vi "小波阈值降噪—优化.vi"(5 "Tab Control":enum32{"None", "Threshold", "Levels"}(tab)=enum."Threshold", 8 "signal out":waveform(dbl)) -> (0 "Denoised Signal":waveform(dbl)(graph)={"t0"=timestamp(0 s since 1904-01-01), "dt"=0.001, "Y"=[]}, 2 "Mean Squared Error":dbl=0.019874592460755663 format="%.2f", 3 "Thresholded Wavelet \nTransform":waveform(dbl)(graph)={"t0"=timestamp(0 s since 1904-01-01), "dt"=0.001, "Y"=[]})   [LabVIEW 2015]
doc: "This LabVIEW VI demonstrates several methods of wavelet-based noise reduction using the Daubechies 4 wavelet. Although it does not require the Signal Processing Toolset, that toolset could be used to extend this demo with other types of wavelets."
uses:
  <vilib>/gmath/NI_Gmath.lvlib
  <vilib>/measure/NI_MABase.lvlib
  <vilib>/Analysis/NI_AALPro.lvlib
panel:
  in  "signal out":waveform(dbl)={"t0"=timestamp(0 s since 1904-01-01), "dt"=0.0, "Y"=[]}
  in  "Threshold":dbl=0.3400000000000002 step=0.01 format="%.2f"
  in  "Keep N Smoothest":i16=10 max=10
  in  "Continuously\nUpdate Signal?":bool
  in  "standard deviation":dbl=0.2 format="%.2f"
  in  "amplitude":dbl=1.0 format="%.2p"
  in  "frequency":dbl=10.0 format="%.2p"
  out "Original (Noise free) signal":waveform(dbl)(graph)={"t0"=timestamp(0 s since 1904-01-01), "dt"=0.001, "Y"=[]}
  out "Signal + Noise":waveform(dbl)(graph)={"t0"=timestamp(0 s since 1904-01-01), "dt"=0.001, "Y"=[]}
  out "Added Noise":waveform(dbl)(graph)={"t0"=timestamp(0 s since 1904-01-01), "dt"=0.001, "Y"=[]}
  in  "sampling info":cluster{"Fs":dbl, "#s":i32}={"Fs"=1000.0, "#s"=1024} {"Fs" format="%.2p"}
  # "Choose a denoising method"
  # "Cut transform values below this threshold?"
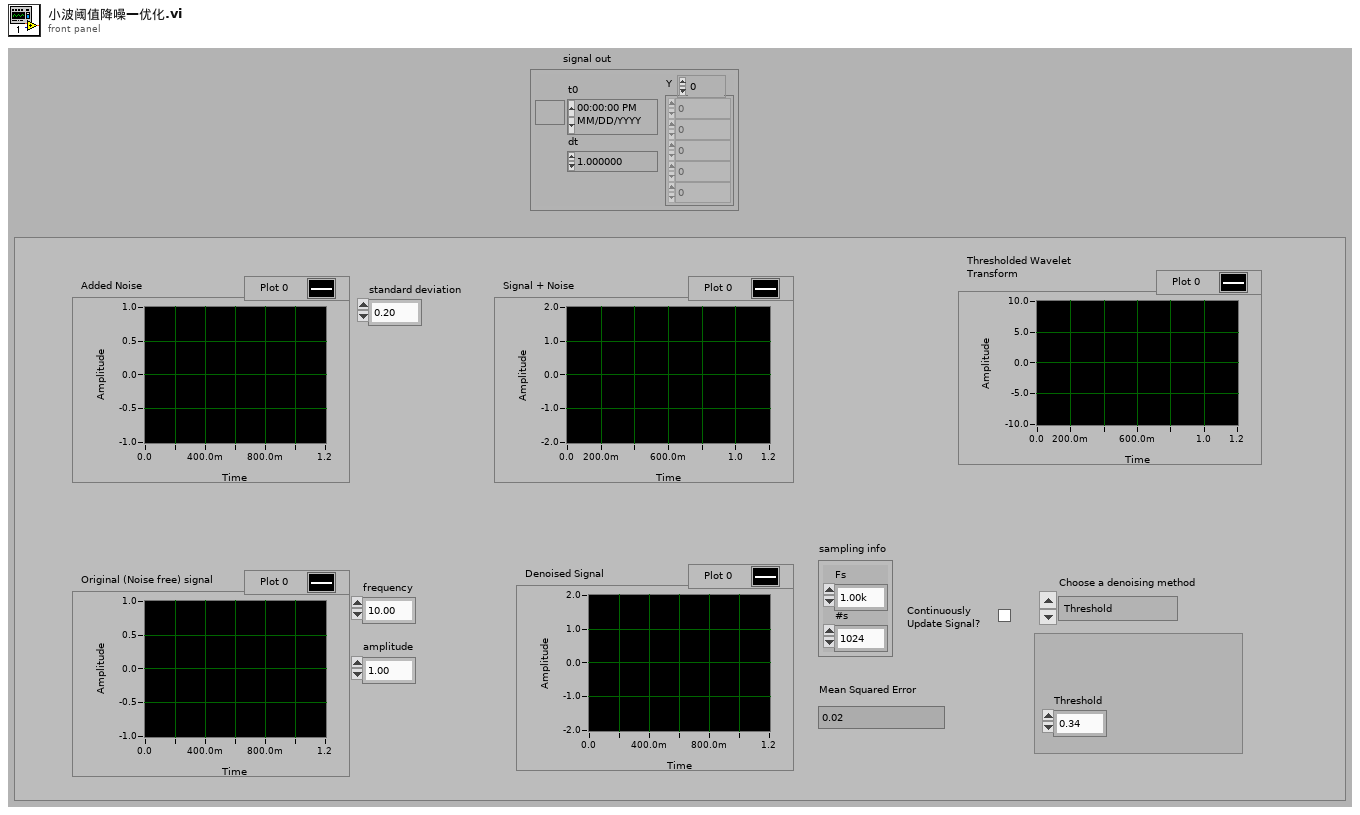
[diagram p1: front panel]
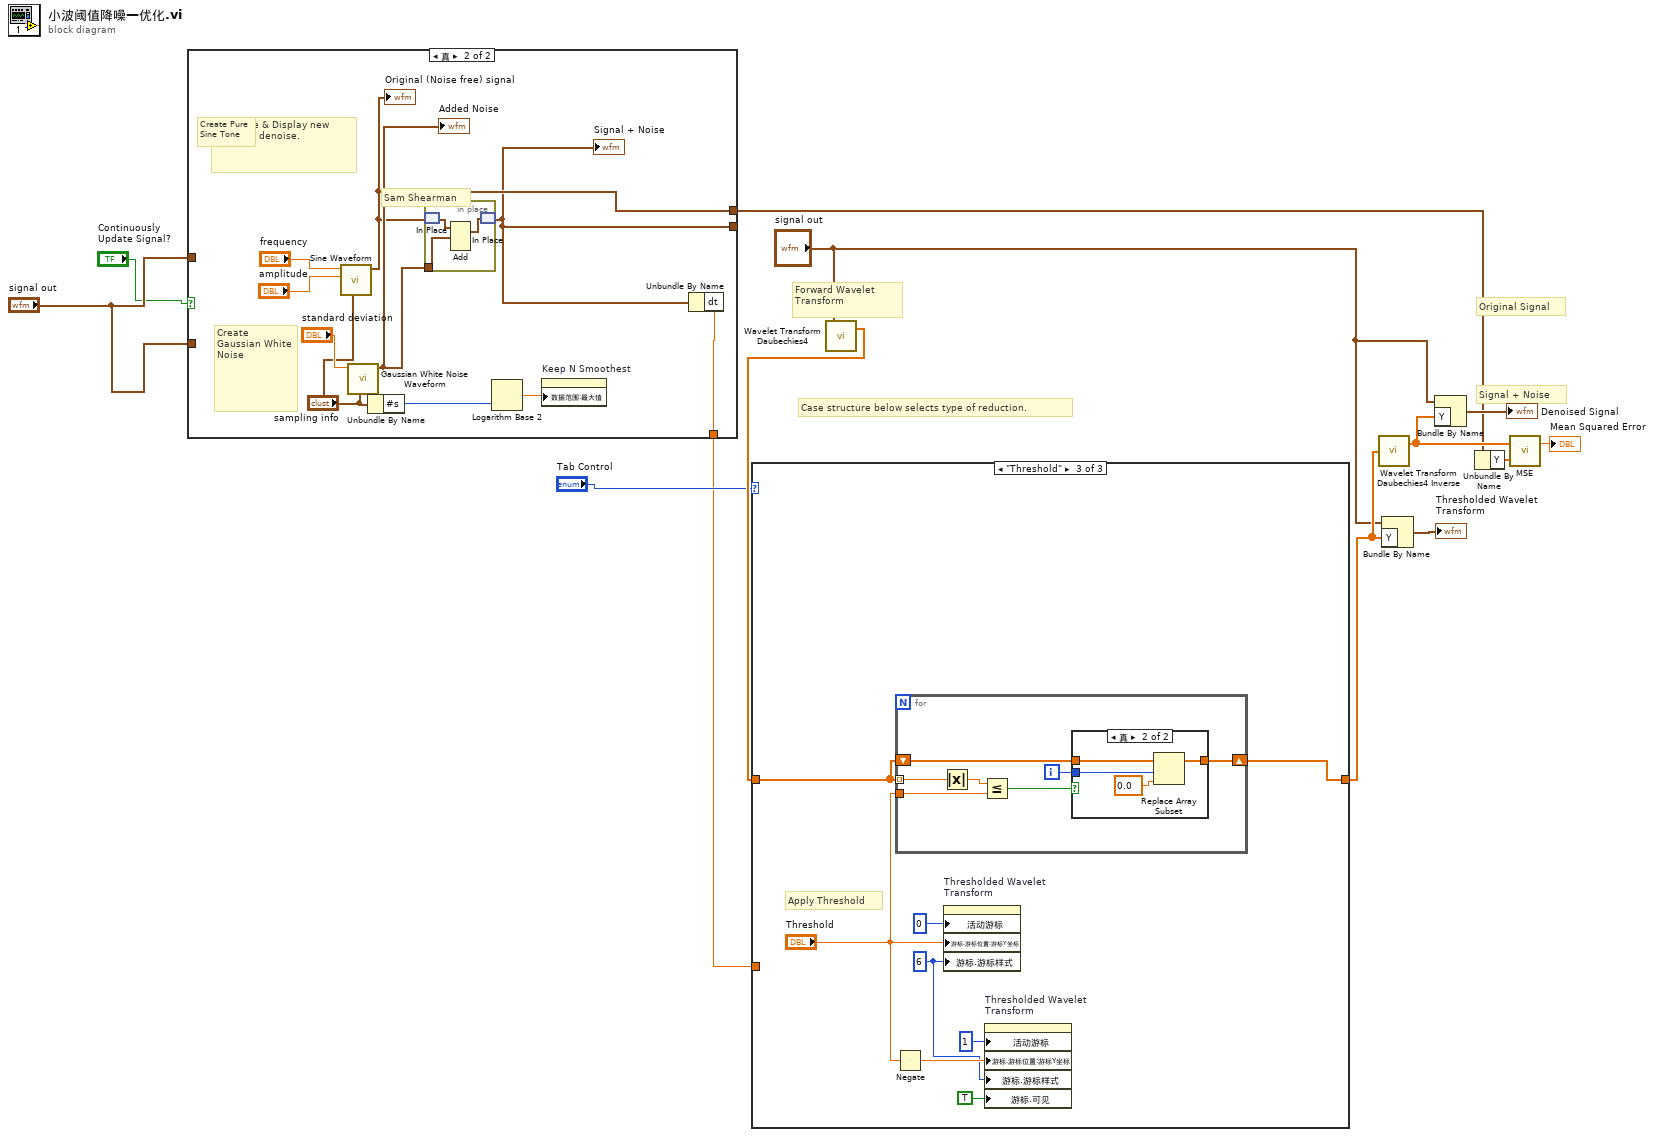
[diagram p0: block diagram]
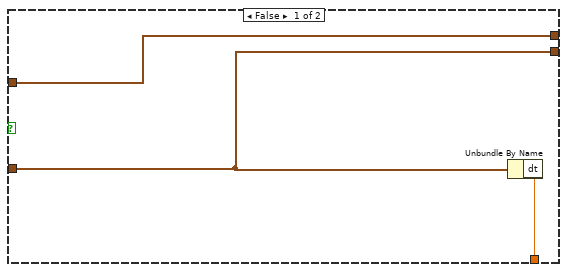
[diagram p2: hidden frame]
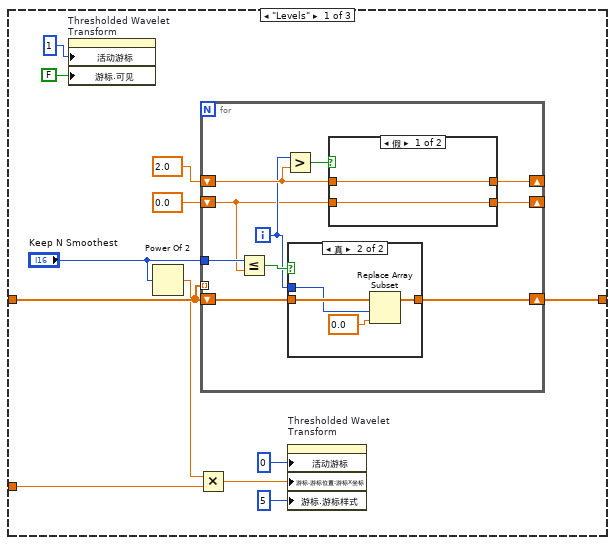
[diagram p3: hidden frame]
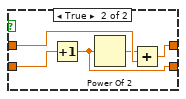
[diagram p5: hidden frame]
diagram:
  # "Case structure below selects type of reduction."
  # "Forward Wavelet Transform"
  # "Sam Shearman"
  # "Signal + Noise"
  # "Original Signal"
  n1 = case shown="真" "Continuously\nUpdate Signal?" {
    tunnel: [w16 w22] -> w4
    tunnel: "signal out" -> [w16 _]
    tunnel: [w15 w18] -> _
    tunnel: "signal out" -> [w15 _]
    tunnel: [w14 w17] -> w2
    frame False {
      n2 = Unbundle By Name(w15) -> ("dt"=w14:dbl)
    }
    frame True {
      # "Generate & Display new signal to denoise."
      # "Create Gaussian White Noise"
      # "Create Pure Sine Tone"
      n3 = call <vilib>:"Sine Waveform.vi"("sampling info"="sampling info", "amplitude"="amplitude", "frequency"="frequency") -> ("signal out"=w22:waveform(dbl))  [unwired: 7 in, 1 out]
      "Original (Noise free) signal" <- w22
      n4 = call <vilib>:"Gaussian White Noise Waveform.vi"("sampling info"="sampling info", "standard deviation"="standard deviation") -> ("signal out"=w23:waveform(dbl))  [unwired: 8 in, 1 out]
      "Added Noise" <- w23
      n5 = Unbundle By Name("sampling info") -> ("#s"=w20:i32)
      n6 = in-place {
        in-place-border: w23 -> [w29]
        n7 = in-place-match #1(w22) -> (w28:waveform(dbl))
        n8 = Add ("Add Waveforms.vi")(1:w29, 2:w28) -> (0:w27:waveform(dbl))  [unwired: 1 in, 1 out]
        n9 = in-place-match #1(w27) -> (w18:waveform(dbl))
      }
      "Signal + Noise" <- w18
      n10 = Logarithm Base 2(1:w20) -> (0:w19:dbl)
      n11 = property on="Keep N Smoothest" class="DigNum (严格)"("数据范围:最大值"=w19) -> ()  [unwired: 2 in, 2 out]
      n12 = Unbundle By Name(w18) -> ("dt"=w17:dbl)
    }
  }
  n13 = call <vilib>:"Wavelet Transform Daubechies4.vi"("X"="signal out") -> ("Wavelet Daubechies4 {X}"=w10:dbl[])  [unwired: 1 out]
  n14 = case shown="\"Threshold\"" "Tab Control" {
    tunnel: w10 -> [w41 w64 w71]
    tunnel: [w40 w64 w72] -> w9
    tunnel: w2 -> [w35 _ _]
    frame "Levels" {
      n15 = property on="Thresholded Wavelet \nTransform" class="WFGraph (严格)"("活动游标"=u32 1 ("Active Cursor"), "游标.可见"=FALSE ("Cursor.Visible")) -> ()  [unwired: 2 in, 2 out]
      n16 = Power Of 2(x="Keep N Smoothest") -> (2^x=w36:dbl)
      n17 = Multiply(x=w36, y=w35) -> (x*y=w34:dbl)
      n18 = for {
        shift-right: [w49] -> _
        shift-left: 2.0 ("y") -> [w50]
        shift-right: [w48] -> _
        shift-left: 0.0 -> [w42]
        tunnel: "Keep N Smoothest" -> [w47]
        shift-right: [w44] -> w40
        shift-left: w41 -> [w45]
        tunnel: w41 -> [_] mode=indexing
        i -> [w43]
        n19 = Less Or Equal?(x=w47, y=w42) -> (x <= y?=w46:bool)
        n20 = Greater?(x=w43, y=w50) -> (0:w51:bool)
        n21 = case shown="真" w46 {
          tunnel: w45 -> [w52 w56]
          tunnel: [w52 w53] -> w44
          tunnel: w43 -> [_ w55]
          frame False {
          }
          frame True {
            n22 = Replace Array Subset(array=w56, new element=0.0 ("new element/subarray"), index=w55) -> (w53:dbl[])
          }
        }
        n23 = case shown="假" w51 {
          tunnel: w50 -> [w57 w63]
          tunnel: [w57 w62] -> w49
          tunnel: w42 -> [w58 w61]
          tunnel: [w58 w59] -> w48
          frame False {
          }
          frame True {
            n24 = Increment(x=w61) -> (x+1=w59:dbl)
            n25 = Power Of 2(x=w59) -> (2^x=w60:dbl)
            n26 = Add(x=w60, y=w63) -> (x+y=w62:dbl)
          }
        }
      }
      n27 = property on="Thresholded Wavelet \nTransform" class="WFGraph (严格)"("活动游标"=u32 0 ("Active Cursor"), "游标.游标位置:游标X坐标"=w34, "游标.游标样式"=u8 5 ("Cursor.Cursor Style")) -> ()  [unwired: 2 in, 2 out]
    }
    frame "None", Default {
      # "No operations"
    }
    frame "Threshold" {
      w66 = u8 6 ("Cursor.Cursor Style")
      # "Apply Threshold"
      n28 = Negate(x="Threshold") -> (-x=w68:dbl)
      n29 = for {
        shift-right: [w78] -> w72
        shift-left: w71 -> [w79]
        tunnel: w71 -> [w77] mode=indexing
        tunnel: "Threshold" -> [w76]
        i -> [w74]
        n30 = Absolute Value(x=w77) -> (abs(x)=w73:dbl)
        n31 = Less Or Equal?(x=w73, y=w76) -> (x <= y?=w75:bool)
        n32 = case shown="真" w75 {
          tunnel: w79 -> [w80 w84]
          tunnel: [w80 w83] -> w78
          tunnel: w74 -> [_ w82]
          frame False {
          }
          frame True {
            n33 = Replace Array Subset(array=w84, new element=0.0 ("New Element/Subarray"), index=w82) -> (w83:dbl[])
          }
        }
      }
      n34 = property on="Thresholded Wavelet \nTransform" class="WFGraph (严格)"("活动游标"=u32 0 ("Active Cursor"), "游标.游标位置:游标Y坐标"="Threshold", "游标.游标样式"=w66) -> ()  [unwired: 2 in, 2 out]
      n35 = property on="Thresholded Wavelet \nTransform" class="WFGraph (严格)"("活动游标"=u32 1 ("Active Cursor"), "游标.游标位置:游标Y坐标"=w68, "游标.游标样式"=w66, "游标.可见"=TRUE ("Cursor.Visible")) -> ()  [unwired: 2 in, 2 out]
    }
  }
  n36 = call <vilib>:"Wavelet Transform Daubechies4 Inverse.vi"("X"=w9) -> ("Wavelet Daubechies4 Inv {X}"=w8:dbl[])  [unwired: 1 out]
  n37 = Bundle By Name(cluster="signal out", "Y"=w9) -> (→"Thresholded Wavelet \nTransform":waveform(dbl))
  n38 = Bundle By Name(cluster="signal out", "Y"=w8) -> (→"Denoised Signal":waveform(dbl))
  n39 = Unbundle By Name(w4) -> ("Y"=w7:dbl[])
  n40 = call <vilib>:"MSE.vi"("X Values"=w7, "Y Values"=w8) -> ("mse"=→"Mean Squared Error":dbl)  [unwired: 1 out]
